vi "ini2JSON (SubVI).vi"(8 "error in (no error)":errorcluster, 10 "section":string, 11 "Refnum in":T1) -> (0 "error out":errorcluster, 2 "JSON":string, 3 "Refnum out":T1)   [LabVIEW 2014]
uses:
  <vilib>/Utility/config.llb/Config Data RefNum.ctl
  <vilib>/Utility/config.llb/Read Key (String).vi
  <vilib>/Utility/config.llb/NI_LVConfig.lvlib
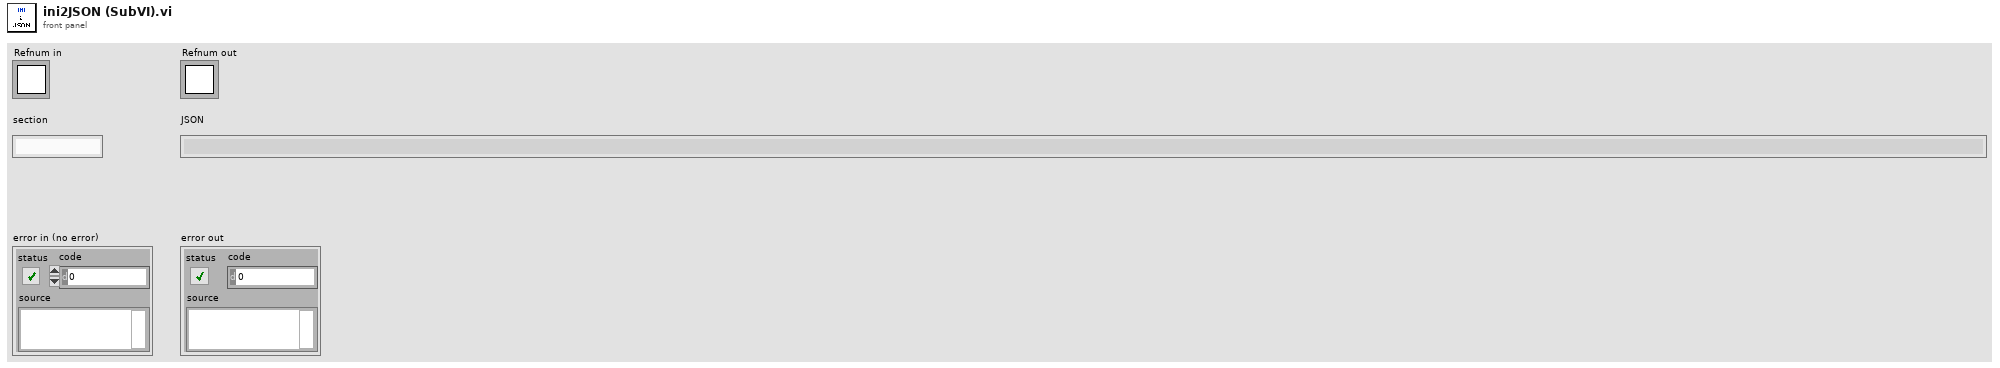
[diagram p1: front panel]
types:
  T1 = typedef "NI_LVConfig.lvlib/Config Data RefNum.ctl" = refnum<k1>
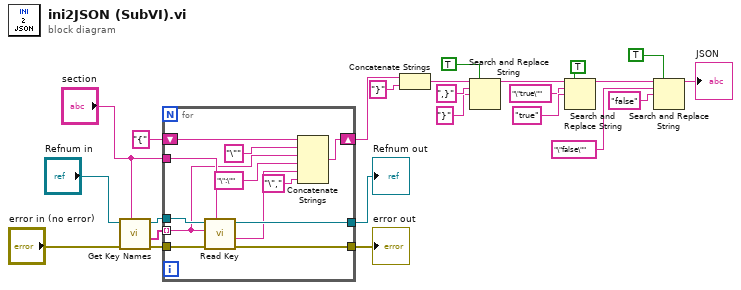
[diagram p0: block diagram]
diagram:
  n1 = call <vilib>:"Get Key Names.vi"("section"="section", "error in (no error)"="error in (no error)", "refnum"="Refnum in") -> ("error out"=w7:errorcluster, "key names"=w5:string[], "refnum out"=w6:T1)  [unwired: 5 in, 1 out]
  n2 = for {
    tunnel: w5 -> [w30] mode=indexing
    tunnel: w6 -> [w36]
    tunnel: w7 -> [w35]
    tunnel: [w32] -> w8
    tunnel: [w34] -> w9
    tunnel: "section" -> [w33]
    shift-right: [w31] -> w12
    shift-left: "{" ("string") -> [w29]
    n3 = call-poly <vilib>:"Read Key.vi"("section"=w33, "error in (no error)"=w35, "key"=w30, "refnum"=w36) -> ("error out"=w32:errorcluster, "value"=w26:string, "refnum out"=w34:T1)  [unwired: 4 in, 1 out]
    n4 = Concatenate Strings(w29, "\"" ("string"), w30, "\":\"" ("string"), w26, "\"," ("string")) -> (w31:string)
  }
  "Refnum out" <- w9
  "error out" <- w8
  n5 = Concatenate Strings(w12, "}" ("string")) -> (w14:string)
  n6 = Search and Replace String(replace all?=TRUE ("replace all? (F)"), input string=w14, search string=",}", replace string="}" ("replace string (\"\")")) -> (result string=w15:string)  [unwired: 4 in, 3 out]
  n7 = Search and Replace String(replace all?=TRUE ("replace all? (F)"), input string=w15, search string="\"true\"", replace string="true" ("replace string (\"\")")) -> (result string=w23:string)  [unwired: 4 in, 3 out]
  n8 = Search and Replace String(replace all?=TRUE ("replace all? (F)"), input string=w23, search string="\"false\"", replace string="false" ("replace string (\"\")")) -> (result string=→"JSON":string)  [unwired: 4 in, 3 out]
